vi "Platinum RTD Ohms to C.vi"(1 "Rt":dbl format="%.1f") -> (0 "Temp (C)":dbl)   [LabVIEW 2010]
panel:
  in  "R0":dbl=1000.0 format="%.1f"
  in  "B":dbl=-6.02e-07 format="%.3e"
  in  "A":dbl=0.00381 format="%.3e"
  # "Temperature Sensors HEL-776/HEL-777 Series, PLATINUM RTD"
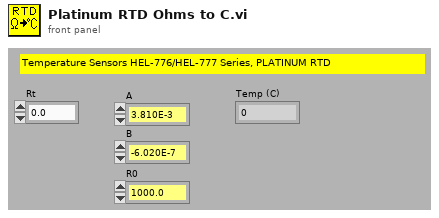
[diagram p1: front panel]
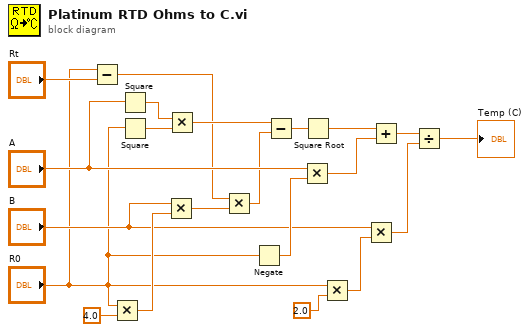
[diagram p0: block diagram]
diagram:
  n1 = Subtract(x="R0", y="Rt") -> (x-y=w3:dbl)
  n2 = Multiply(x="R0", y=4.0) -> (x*y=w8:dbl)
  n3 = Square(x="A") -> (x^2=w14:dbl)
  n4 = Square(x="R0") -> (x^2=w15:dbl)
  n5 = Multiply(x="B", y=w8) -> (x*y=w6:dbl)
  n6 = Multiply(x=w14, y=w15) -> (x*y=w13:dbl)
  n7 = Multiply(x=w3, y=w6) -> (x*y=w2:dbl)
  n8 = Negate(x="R0") -> (-x=w17:dbl)
  n9 = Subtract(x=w13, y=w2) -> (x-y=w1:dbl)
  n10 = Multiply(x="A", y=w17) -> (x*y=w12:dbl)
  n11 = Square Root(x=w1) -> (sqrt(x)=w10:dbl)
  n12 = Multiply(x="R0", y=2.0) -> (x*y=w20:dbl)
  n13 = Multiply(x="B", y=w20) -> (x*y=w18:dbl)
  n14 = Add(x=w10, y=w12) -> (x+y=w11:dbl)
  n15 = Divide(x=w11, y=w18) -> (x/y=→"Temp (C)":dbl)
